vi "Get Count.vi"(8 "error in (no error)":errorcluster, 11 "Core Channel Configuration in":refnum<class "Core Channels Configuration.lvclass">) -> (0 "error out":errorcluster, 2 "count":i32, 3 "Core Channel Configuration out":refnum<class "Core Channels Configuration.lvclass">)   [LabVIEW 2017, in "DSF Core.lvlib" / "Core Channels Configuration.lvclass"]
uses:
  Core Channels Configuration.lvclass
  Core Channels Configuration.lvclass/Core Channels Configuration.ctl
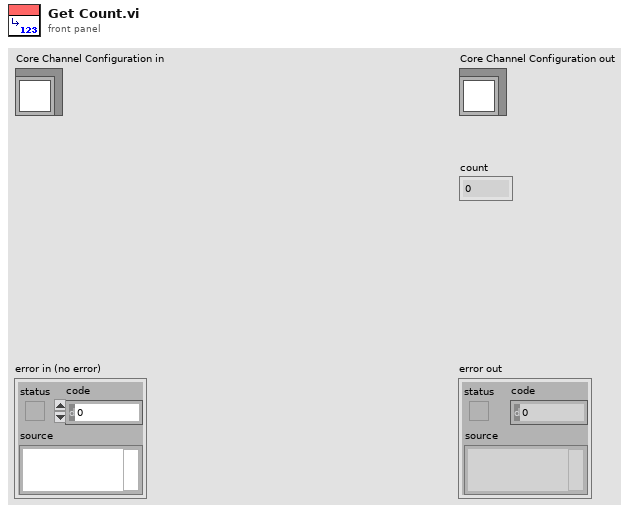
[diagram p1: front panel]
types:
  T1 = typedef "DSF Core.lvlib/Core Channels Configuration.lvclass/Configuration.ctl" = cluster{"name":string, "units":string, "engine data type":T2, "string data type":T2, "string offset":u64}
  T2 = typedef "DSF Core.lvlib/DSF Data Type.ctl" = enum8{"Bool", "SGL", "DBL", "I8", "I16", "I32", "I64", "U8", "U16", "U32", "U64"}
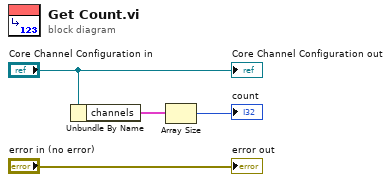
[diagram p0: block diagram]
diagram:
  n1 = Unbundle By Name("Core Channel Configuration in") -> ("channels"=w4:T1[])
  n2 = Array Size(array=w4) -> (size(s)=→"count":i32)
  "error out" <- "error in (no error)"
  "Core Channel Configuration out" <- "Core Channel Configuration in"
